vi "Calculate nPixCamera and nAT per B.vi"(11 "Scan Parameters":T1={"# Scan"={"#Ascan"=400, "#Bscan"=400}, "# Rpt"={"#ARpt"=1, "#BRpt"=1}, "Aline Rate"=2, "# Extra"={"# ARpt_extra"=5, "#Brtn_extra"=60}} {"Aline Rate" items=["76 KHz", "146 KHz", "76 KHz", "28 KHz", "10 KHz"]}) -> (1 "initialized array":u16[][](array[numeric]), 2 "nAT per B":i32, 3 "nPix Camera Out":i32=2048)   [LabVIEW 2017]
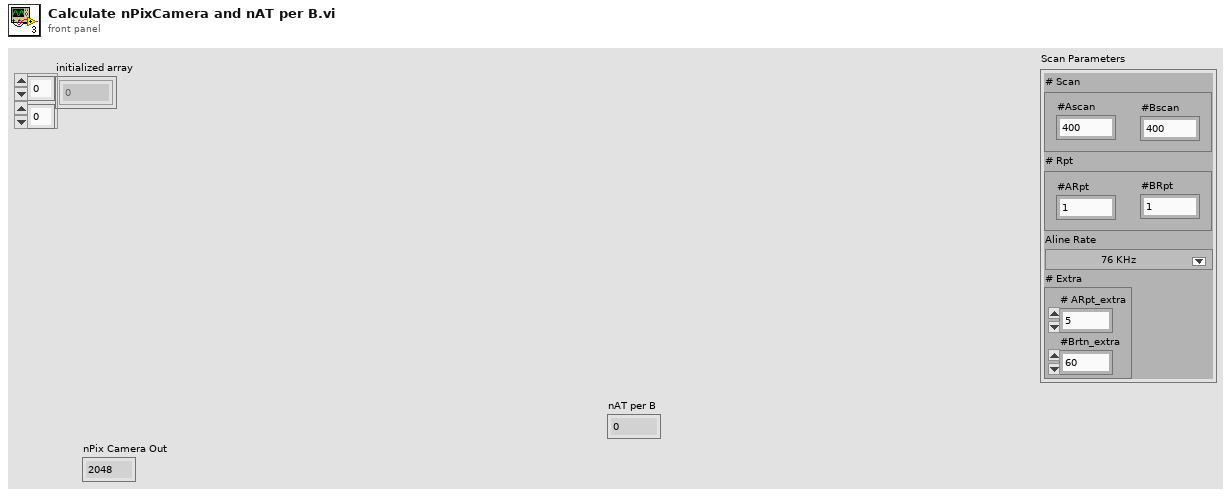
[diagram p1: front panel]
types:
  T1 = cluster{"# Scan":cluster{"#Ascan":i32, "#Bscan":i32}, "# Rpt":cluster{"#ARpt":i32, "#BRpt":i32}, "Aline Rate":u16, "# Extra":cluster{"# ARpt_extra":i32, "#Brtn_extra":i32}}
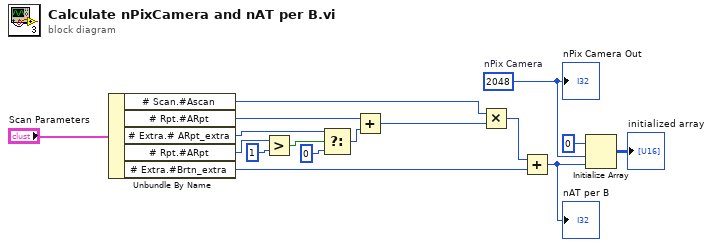
[diagram p0: block diagram]
diagram:
  w9 = 2048  # nPix Camera
  n1 = Unbundle By Name("Scan Parameters") -> ("# Scan.#Ascan"=w5:i32, "# Rpt.#ARpt"=w4:i32, "# Extra.# ARpt_extra"=w3:i32, "# Rpt.#ARpt"=w2:i32, "# Extra.#Brtn_extra"=w1:i32)
  n2 = Greater?(x=w2, y=1) -> (0:w15:bool)
  n3 = Select(t=w3, s=w15, f=0) -> (s? t:f=w13:i32)
  n4 = Add(x=w4, y=w13) -> (x+y=w12:i32)
  n5 = Multiply(x=w5, y=w12) -> (x*y=w11:i32)
  n6 = Add(x=w11, y=w1) -> (x+y=w8:i32)
  "nAT per B" <- w8
  n7 = Initialize Array(u16 0 ("element"), w9, w8) -> (→"initialized array":u16[][])
  "nPix Camera Out" <- w9
